vi "error_messages_global.vi"() -> ()   [LabVIEW 2010]
panel:
  in  "error messages?":bool
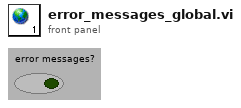
[diagram p1: front panel]
diagram:
